vi "test_UPDtxrxLoopback.vi"() -> ()   [LabVIEW 2020]
uses:
  <instrlib>/AIM GmbH/_AIM 664/_controls/comm_verification_rx.ctl
  <instrlib>/AIM GmbH/_AIM 664/_controls/comm_config_vl_tx.ctl
  <instrlib>/AIM GmbH/_AIM 664/_controls/comm_udp_rx.ctl
  <instrlib>/AIM GmbH/_AIM 664/helpers/EthFrameManagement/controls/arinc664_mac_src_info.ctl
  <instrlib>/AIM GmbH/_AIM 664/_controls/comm_udp_tx.ctl
  <instrlib>/AIM GmbH/_AIM 664/bsp/Controls/IrigTime.ctl
  <instrlib>/AIM GmbH/_AIM 664/bsp/Fdx Create Session (Tx-UDP Port-Oriented).vi
  <instrlib>/AIM GmbH/_AIM 664/bsp/Fdx Create Session (Rx-VL-Oriented).vi
  <instrlib>/AIM GmbH/_AIM 664/bsp/Receive/FdxCreateRxVL.vi
  <instrlib>/AIM GmbH/_AIM 664/bsp/Transmit/FdxCreateTxVL.vi
  <instrlib>/AIM GmbH/_AIM 664/bsp/Fdx Create UDP Port (RX-CommPort).vi
  <instrlib>/AIM GmbH/_AIM 664/bsp/Fdx Create UDP Port (TX-CommPort).vi
  <instrlib>/AIM GmbH/_AIM 664/bsp/Fdx Start (Rx).vi
  <instrlib>/AIM GmbH/_AIM 664/bsp/Fdx Stop (Rx).vi
  <instrlib>/AIM GmbH/_AIM 664/bsp/Fdx Start (Tx).vi
  <instrlib>/AIM GmbH/_AIM 664/bsp/Fdx Stop (Tx).vi
  <instrlib>/AIM GmbH/_AIM 664/AIM664LV.lvlib
  <instrlib>/AIM GmbH/_AIM 664/helpers/EthFrameManagement/EthFrameManagement.lvlib
panel:
  out "time stamp":timestamp
  out "timestamp s":dbl
  out "ul_ErrorInfo":u32
  out "ul_MsgSize":u32
  out "IrigTime":T1
  out "MsgCount":u32
  out "IndexCycleCount":u32
  out "CurrentIndex":u32
  in  "stop":bool
  out "TxStatus":T2 {"TransmitMode" items=["FDX_TX_GENERIC", "FDX_TX_REPLAY", "FDX_TX_INDIVIDUAL"]; "TxStatus" items=["FDX_STAT_STOP", "FDX_STAT_RUN", "FDX_STAT_ERROR", "FDX_STAT_WAIT_F_TRIG"]}
  out "GlobalStat Out":T3
  out "MsgErrorCount":u32
  out "RxStatus":u32
  out "Info":u32
  out "MsgRead":u32
  out "ReadBuffer":u8[](array[numeric]) format="%.0x"
  out "error out":errorcluster
  out "retries":i32
  in  "mst th (1)":u32=1
  out "Buf":u8[](array[numeric]) format="%.0x"
  in  "Buf Lenght":i32=512
  in  "CommPort Config":T4={"PortType"=enum."FDX_UDP_SAMPLING", "partitionID"=1, "SubVlId"=1, "UdpSrcPort"=24, "UdpDstPort"=23, "SampleRateMs"=64.0, "UdpNumBufMessages"=1, "UdpMaxMessageSize"=512}
  in  "VlTx":T5={"domainID"=1, "sideID"=1, "locationID"=1, "interfaceID"=1}
  in  "CommPort Config":T6={"PortType"=enum."FDX_UDP_SAMPLING", "SubVIId"=1, "domainID"=1, "sideID"=1, "locationID"=1, "partitionID"=1, "UdpSrcPort"=24, "UdpDstPort"=23, "UdpNumBufMessages"=1, "UdpMaxMessageSize"=512, "UdpSamplingRate"=0} {"partitionID" format="%.0b"}
  in  "tx VL":T7={"VlId"=60, "NumOfSubVl"=4, "rate ms [Bag]"=64, "domainID"=1, "sideID"=1, "locationID"=1, "interfaceID"=1, "NetSelect"=3, "Skew"=0, "MaxFrameLength"=1518, "FrameBufferSize"=0} {"NetSelect" items=["FDX_TX_FRAME_DLY_A"=0, "FDX_TX_FRAME_DLY_B"=1, "FDX_TX_FRAME_BOTH "=3, "FDX_TX_FRAME_ONLY_A"=4, "FDX_TX_FRAME_ONLY_B "=5]; "interfaceID" format="%.0b"}
  in  "rx VL":T8={"VlId"=60, "VLRange"=1, "VerificationMode"=0, "Bag"=0, "Jitter"=0, "MaxFrameLength"=0, "MaxSkew"=0, "VLBufSize"=32768, "FilterMode"=0, "FilterPosition"=0, "Padding"=0, "FilterMask"=0, "FilterData"=0, "MinFrameLength"=0} {"FilterMode" items=["FDX_RX_VL_FLT_DIS", "FDX_RX_VL_FLT_ENA ", "FDX_RX_VL_FLT_ENA_INV"]; "VLBufSize" format="%.0x"; "MaxFrameLength" format="%.0x"; "VerificationMode" items=["FDX_RX_VL_CHECK_ENA_DEFAULT"=65535, "FDX_RX_VL_CHECK_REDMAM"=16, "DX_RX_VL_CHECK_TRAFIC"=8, "FDX_RX_VL_CHECK_FRAMESIZE"=4, "FDX_RX_VL_CHECK_SNINTEG"=2, "FDX_RX_VL_CHECK_INVPAC"=1, "FDX_RX_VL_CHECK_DISA"=0]}
  in  "rx port":u32
  in  "tx port":u32
  in  "rx board":u32=1
  in  "tx board":u32
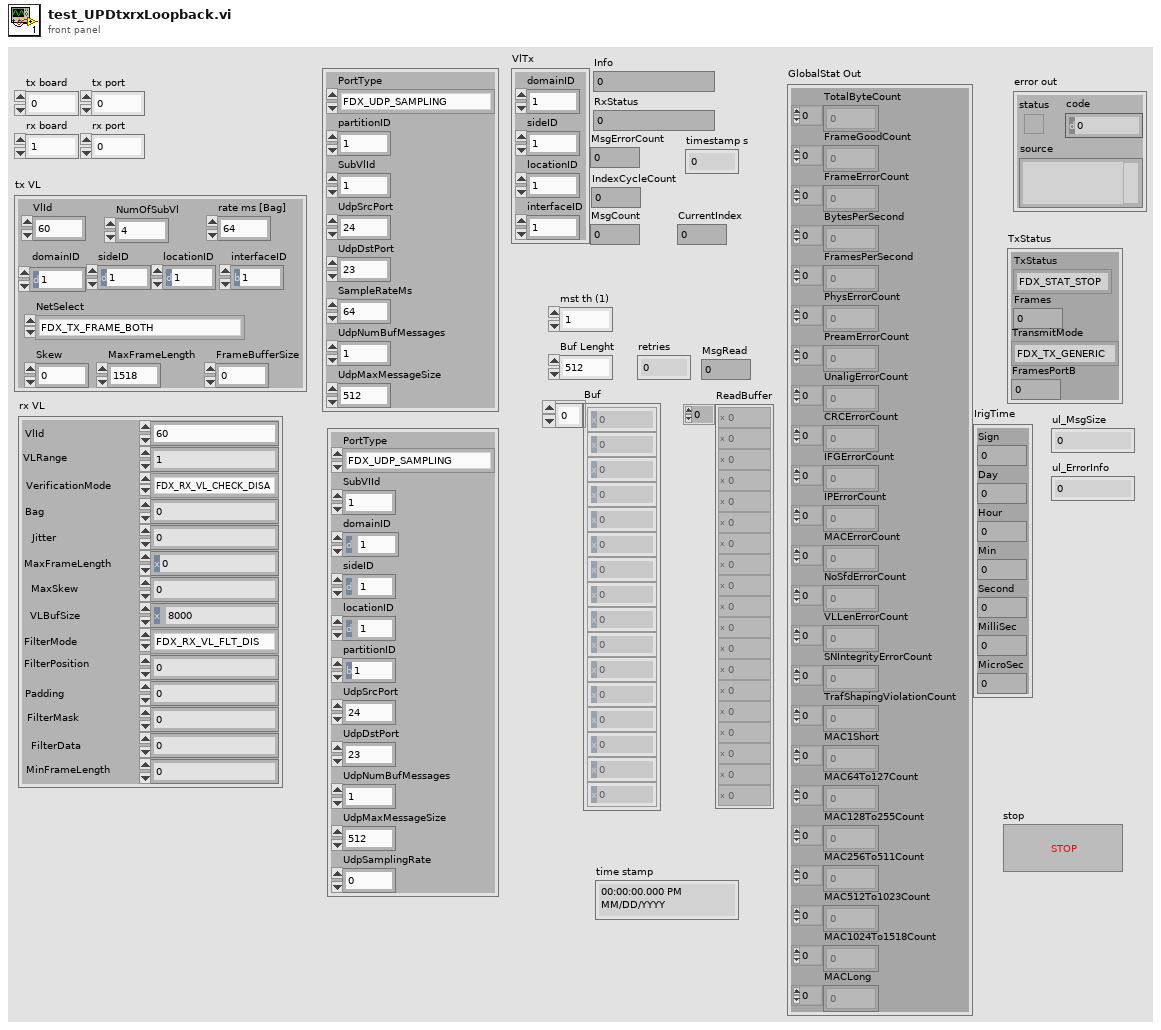
[diagram p1: front panel]
types:
  T1 = typedef "AIM664LV.lvlib/IrigTime.ctl" = cluster{"Sign":i32, "Day":u32, "Hour":u32, "Min":u32, "Second":u32, "MilliSec":u32, "MicroSec":u32}
  T2 = cluster{"TxStatus":u32, "Frames":u32, "TransmitMode":u32, "FramesPortB":u32}
  T3 = cluster{"TotalByteCount":u32[], "FrameGoodCount":u32[], "FrameErrorCount":u32[], "BytesPerSecond":u32[], "FramesPerSecond":u32[], "PhysErrorCount":u32[], "PreamErrorCount":u32[], "UnaligErrorCount":u32[], "CRCErrorCount":u32[], "IFGErrorCount":u32[], "IPErrorCount":u32[], "MACErrorCount":u32[], "NoSfdErrorCount":u32[], "VLLenErrorCount":u32[], "SNIntegrityErrorCount":u32[], "TrafShapingViolationCount":u32[], "MAC1Short":u32[], "MAC64To127Count":u32[], "MAC128To255Count":u32[], "MAC256To511Count":u32[], "MAC512To1023Count":u32[], "MAC1024To1518Count":u32[], "MACLong":u32[]}
  T4 = typedef "AIM664LV.lvlib/comm_udp_tx.ctl" = cluster{"PortType":enum16{"FDX_UDP_SAMPLING", "FDX_UDP_QUEUING"}, "partitionID":u8, "SubVlId":u8, "UdpSrcPort":u16, "UdpDstPort":u16, "SampleRateMs":dbl, "UdpNumBufMessages":u32, "UdpMaxMessageSize":u32}
  T5 = typedef "EthFrameManagement.lvlib/arinc664_mac_src_info.ctl" = cluster{"domainID":u8, "sideID":u8, "locationID":u8, "interfaceID":u8}
  T6 = typedef "AIM664LV.lvlib/comm_udp_rx.ctl" = cluster{"PortType":enum16{"FDX_UDP_SAMPLING", "FDX_UDP_QUEUING"}, "SubVIId":u32, "domainID":u8, "sideID":u8, "locationID":u8, "partitionID":u8, "UdpSrcPort":u16, "UdpDstPort":u16, "UdpNumBufMessages":u32, "UdpMaxMessageSize":u32, "UdpSamplingRate":u32}
  T7 = typedef "AIM664LV.lvlib/comm_config_vl_tx.ctl" = cluster{"VlId":u16, "NumOfSubVl":u16, "rate ms [Bag]":u32, "domainID":u8, "sideID":u8, "locationID":u8, "interfaceID":u8, "NetSelect":u32, "Skew":u32, "MaxFrameLength":u32, "FrameBufferSize":u32}
  T8 = typedef "AIM664LV.lvlib/comm_verification_rx.ctl" = cluster{"VlId":u16, "VLRange":u32, "VerificationMode":u32, "Bag":u32, "Jitter":u32, "MaxFrameLength":u32, "MaxSkew":u32, "VLBufSize":u32, "FilterMode":u32, "FilterPosition":u32, "Padding":u32, "FilterMask":u32, "FilterData":u32, "MinFrameLength":u32}
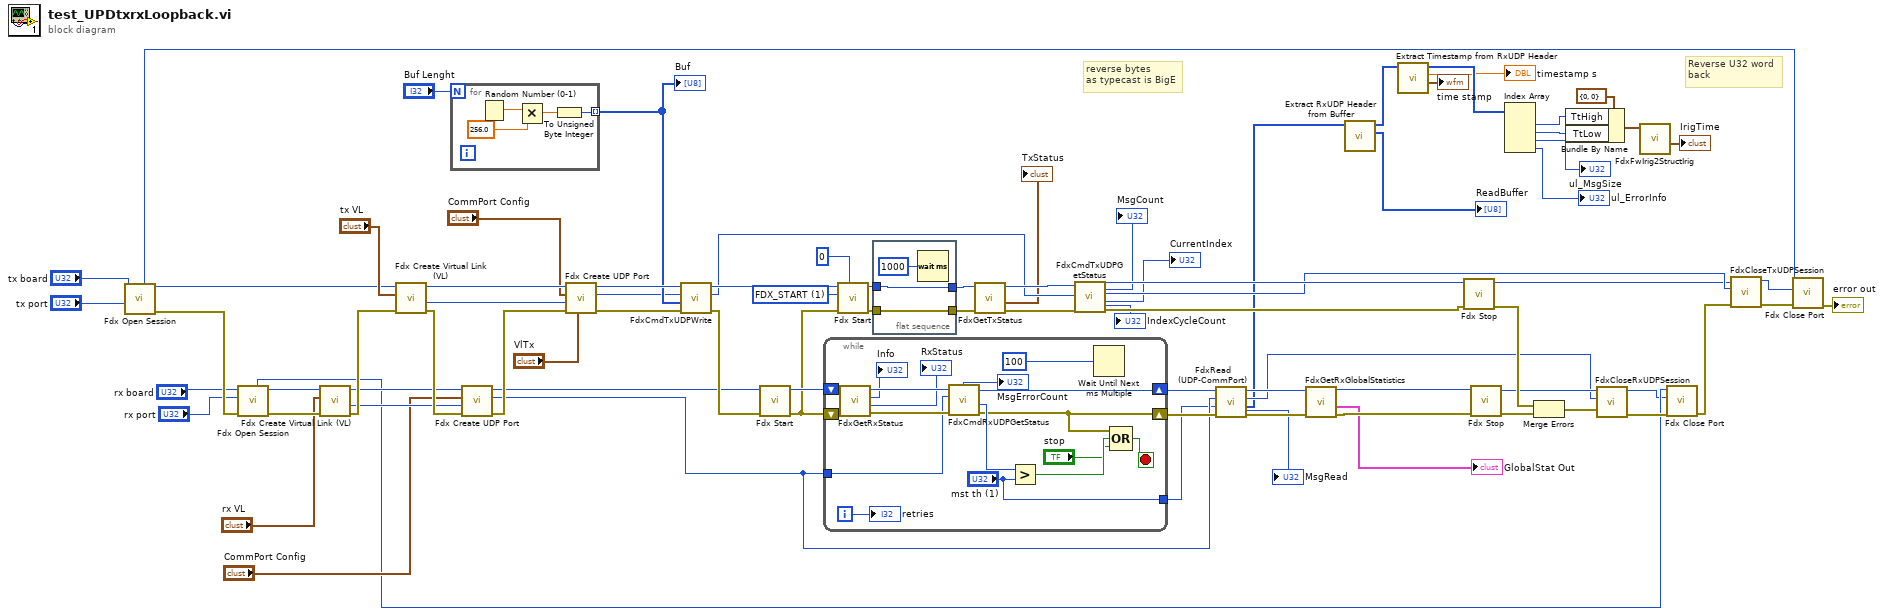
[diagram p0: block diagram]
diagram:
  w15 = 1 items=["FDX_STOP", "FDX_START", "FDX_START_TRG", "FDX_START_TIME"] ("StartMode")
  # "Reverse U32 word\nback"
  # "reverse bytes\nas typecast is BigE"
  n1 = call-poly <instrlib>:"Fdx Open Session.vi"("port"="tx port", "board"="tx board") -> ("error out"=w83:errorcluster, "port handle out"=w73:u32, "InstrumentHandle_board out"=w32:u32)  [unwired: 5 in, 2 out]
  n2 = call-poly <instrlib>:"Fdx Open Session.vi"("error in (no error)"=w83, "port"="rx port", "board"="rx board") -> ("error out"=w78:errorcluster, "InstrumentHandle_port out"=w76:u32, "InstrumentHandle_board out"=w31:u32)  [unwired: 3 in, 3 out]
  n3 = call-poly <instrlib>:"Fdx Create Virtual Link (VL).vi"("error in (no error)"=w78, "VL Config"="rx VL", "InstrumentHandle_port in"=w76) -> ("error out"=w74:errorcluster, "VlId"=w65:u16, "InstrumentHandle_port out"=w69:u32)  [unwired: 6 in]
  n4 = call-poly <instrlib>:"Fdx Create Virtual Link (VL).vi"("error in (no error)"=w74, "VL Config"="tx VL", "InstrumentHandle in"=w73) -> ("error out"=w72:errorcluster, "VlId"=w66:u16, "InstrumentHandle out"=w70:u32)  [unwired: 6 in]
  n5 = for {
    N: "Buf Lenght" -> [_]
    tunnel: [w84] -> w60 mode=indexing
    n6 = Random Number (0-1)() -> (number: 0 to 1=w87:dbl)
    n7 = Multiply(x=w87, y=256.0) -> (x*y=w85:dbl)
    n8 = To Unsigned Byte Integer(number=w85) -> (unsigned 8bit integer=w84:u8)
  }
  "Buf" <- w60
  n9 = call-poly <instrlib>:"Fdx Create UDP Port.vi"("error in"=w72, "VlId"=w65, "CommPort Config"="CommPort Config", "port handle in"=w69) -> ("error out"=w71:errorcluster, "commPort handle out"=w50:u32, "port handle out"=w57:u32)  [unwired: 4 in, 1 out]
  n10 = call-poly <instrlib>:"Fdx Create UDP Port.vi"("VlTx"="VlTx", "error in"=w71, "VlId"=w66, "CommPort Config"="CommPort Config", "port handle in"=w70) -> ("error out"=w61:errorcluster, "commPort handle out"=w59:u32, "port handle out"=w62:u32)  [unwired: 3 in, 1 out]
  n11 = call <instrlib>:"FdxCmdTxUDPWrite.vi"("error in"=w61, "Data"=w60, "UdpHandle"=w59, "InstrumentHandle"=w62) -> ("error out"=w58:errorcluster, "UdpHandleOut"=w38:u32, "InstrumentHandle"=w54:u32)  [unwired: 4 in, 1 out]
  n12 = call-poly <instrlib>:"Fdx Start.vi"("error in"=w58, "InstrumentHandle_port in"=w57) -> ("error out"=w55:errorcluster, "InstrumentHandle_port out"=w56:u32)  [unwired: 8 in]
  n13 = while {
    shift-right: [w95] -> w51
    shift-left: w55 -> [w101]
    tunnel: w50 -> [w94]
    tunnel: ["mst th (1)"] -> w49
    shift-right: [w92] -> w48
    shift-left: w56 -> [w104]
    i -> [w99]
    stop <- w96 stop-if-true
    n14 = call <instrlib>:"FdxGetRxStatus.vi"("error in"=w101, "InstrumentHandle_port in"=w104) -> ("error out"=w102:errorcluster, "RxStatus"=→"RxStatus":u32, "Info"=→"Info":u32, "InstrumentHandle_port out"=w103:u32)  [unwired: 6 in]
    n15 = call <instrlib>:"FdxCmdRxUDPGetStatus.vi"("error in"=w102, "UdpHandle"=w94, "InstrumentHandle_port"=w103) -> ("error out"=w95:errorcluster, "MsgCount"=w100:u32, "InstrumentHandle_port"=w92:u32, "MsgErrorCount"=→"MsgErrorCount":u32)  [unwired: 4 in, 1 out]
    n16 = Greater?(x=w100, y="mst th (1)") -> (0:w97:bool)
    n17 = Wait Until Next ms Multiple(millisecond multiple=u32 100) -> ()  [unwired: 1 out]
    n18 = Compound Arithmetic op=OR(w95, w97, "stop") -> (w96:bool)
    "retries" <- w99
  }
  n19 = call-poly <instrlib>:"Fdx Start.vi"("TransmitTime"=u32 0, "error in"=w55, "StartMode"=w15, "InstrumentHandle_port in"=w54) -> ("error out"=w21:errorcluster, "InstrumentHandle_port out"=w22:u32)  [unwired: 6 in]
  n20 = flat-sequence {
    tunnel: w22 -> [w106]
    tunnel: w21 -> [w105]
    tunnel: [w106] -> w20
    tunnel: [w105] -> w19
    frame #0 {
      n21 = Wait (ms)(milliseconds to wait=u32 1000) -> ()  [unwired: 1 out]
    }
  }
  n22 = call <instrlib>:"FdxGetTxStatus.vi"("error in"=w19, "InstrumentHandle_port"=w20) -> ("error out"=w40:errorcluster, "TxStatus"=→"TxStatus":T2, "InstrumentHandle_port"=w39:u32)  [unwired: 7 in]
  n23 = call <instrlib>:"FdxCmdTxUDPGetStatus.vi"("error in"=w40, "UdpHandle"=w38, "InstrumentHandle"=w39) -> ("error out"=w37:errorcluster, "CurrentIndex"=→"CurrentIndex":u32, "UdpHandleOut"=w35:u32, "InstrumentHandle"=w36:u32, "IndexCycleCount"=→"IndexCycleCount":u32, "MsgCount"=→"MsgCount":u32)  [unwired: 3 in]
  n24 = call <instrlib>:"FdxRead (UDP-CommPort).vi"("error in"=w51, "MsgCount"=w49, "UdpHandle"=w50, "InstrumentHandle_port"=w48) -> ("error out"=w47:errorcluster, "ReadBuffer"=w13:u8[], "UdpHandle  Out"=w26:u32, "InstrumentHandle_port"=w27:u32, "MsgRead"=→"MsgRead":u32)  [unwired: 3 in]
  n25 = call <instrlib>:"FdxGetRxGlobalStatistics.vi"("error in"=w47, "InstrumentHandle_port in"=w27) -> ("error out"=w46:errorcluster, "GlobalStat Out"=→"GlobalStat Out":T3, "InstrumentHandle_port out"=w28:u32)  [unwired: 7 in]
  n26 = call "Extract RxUDP Header from Buffer.vi"("ReadBuffer in"=w13) -> ("Udp Message"=→"ReadBuffer":u8[], "Header"=w4:u32[])  [unwired: 9 in]
  n27 = call "Extract Timestamp from RxUDP Header.vi"("header in"=w4) -> ("time stamp"=→"time stamp":timestamp, "timestamp s"=→"timestamp s":dbl, "header out"=w3:u32[])  [unwired: 8 in]
  n28 = call-poly <instrlib>:"Fdx Stop.vi"("error in"=w37, "InstrumentHandle_port in"=w36) -> ("error out"=w44:errorcluster, "InstrumentHandle_port out"=w34:u32)  [unwired: 8 in]
  n29 = call-poly <instrlib>:"Fdx Stop.vi"("error in"=w46, "InstrumentHandle_port in"=w28) -> ("error out"=w53:errorcluster, "InstrumentHandle_port out"=w29:u32)  [unwired: 8 in]
  n30 = Index Array(array=w3) -> (element #1=w10:u32, element #2=w9:u32, element #3=→"ul_MsgSize":u32, element #4=→"ul_ErrorInfo":u32)  [unwired: 4 in]
  n31 = Merge Errors(w44, w53) -> (w45:errorcluster)
  n32 = Bundle By Name(cluster=cluster{"TtHigh":u32, "TtLow":u32} {"TtHigh"=0, "TtLow"=0} ("FwIrigTime"), "TtHigh"=w10, "TtLow"=w9) -> (w11:cluster{"TtHigh":u32, "TtLow":u32})
  n33 = call <instrlib>:"FdxCloseRxUDPSession.vi"("error in"=w45, "UdpHandle"=w26, "InstrumentHandle_port"=w29) -> ("error out"=w52:errorcluster, "InstrumentHandle_port"=w30:u32)  [unwired: 7 in]
  n34 = call <instrlib>:"FdxFwIrig2StructIrig.vi"("FwIrigTime"=w11) -> ("IrigTime"=→"IrigTime":T1)  [unwired: 9 in, 1 out]
  n35 = call <instrlib>:"Fdx Close Port.vi"("error in"=w52, "InstrumentHandle_port in"=w30, "InstrumentHandle_board in"=w31) -> ("error out"=w43:errorcluster)  [unwired: 7 in, 1 out]
  n36 = call <instrlib>:"FdxCloseTxUDPSession.vi"("error in"=w43, "UdpHandle"=w35, "InstrumentHandle"=w34) -> ("error out"=w42:errorcluster, "InstrumentHandle"=w33:u32)  [unwired: 7 in]
  n37 = call <instrlib>:"Fdx Close Port.vi"("error in"=w42, "InstrumentHandle_port in"=w33, "InstrumentHandle_board in"=w32) -> ("error out"=→"error out":errorcluster)  [unwired: 7 in, 1 out]
